vi "Execute Change Boolean Image.vi"(6 "Mouse Position":T1, 8 "User VI Ref":refnum<vi>, 9 "Menu Item Tag Suffix":string, 10 "Remaining Items":refnum<vi>[](array[refnum]), 11 "Affected Items":cluster{"Controls":refnum<vi>[]}) -> (0 "Fail transaction?":bool)   [LabVIEW 2021]
doc: "This VI will set a Boolean type that is input to the control's tag and stays persistent. It marks the data that is used in future application when changing themes.\n\n<b>Original</b>:This VI is part of a plug-in for modifying the LabVIEW shortcut menus. This is the execute VI which is called when the shortcut menu is chosen by the user. It performs the action of the selected menu item."
uses:
  Material-Scheme/Material-Scheme.lvclass
  <vilib>/Utility/miscctls.llb/LVPositionTypeDef.ctl
  Material SubVIs/Material SubVIs.lvlib
panel:
  # "All controls on this panel except \"Affected Items\" have been locked to prevent accidental edits. Changing the control names or types, other than the elements of the \"Affected Items\" cluster will make the VI unusable as a menu plugin.\n\nSee Context Help for each control for details about its use."
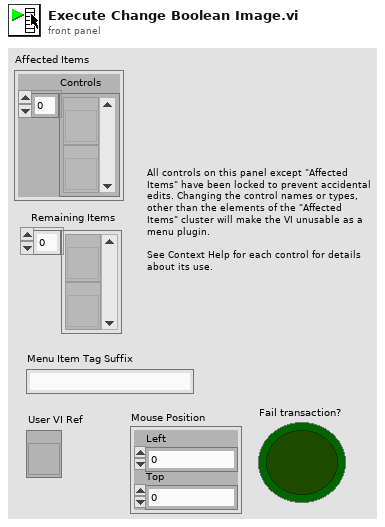
[diagram p1: front panel]
types:
  T1 = typedef "LVPositionTypeDef.ctl" = cluster{"Left":i32, "Top":i32}
  T2 = enum32{"invalid VI type", "Standard VI", "Control VI", "Global VI", "Polymorphic VI", "Configuration VI", "SubSystem", "Facade VI", "Method VI", "Statechart Diagram VI"}
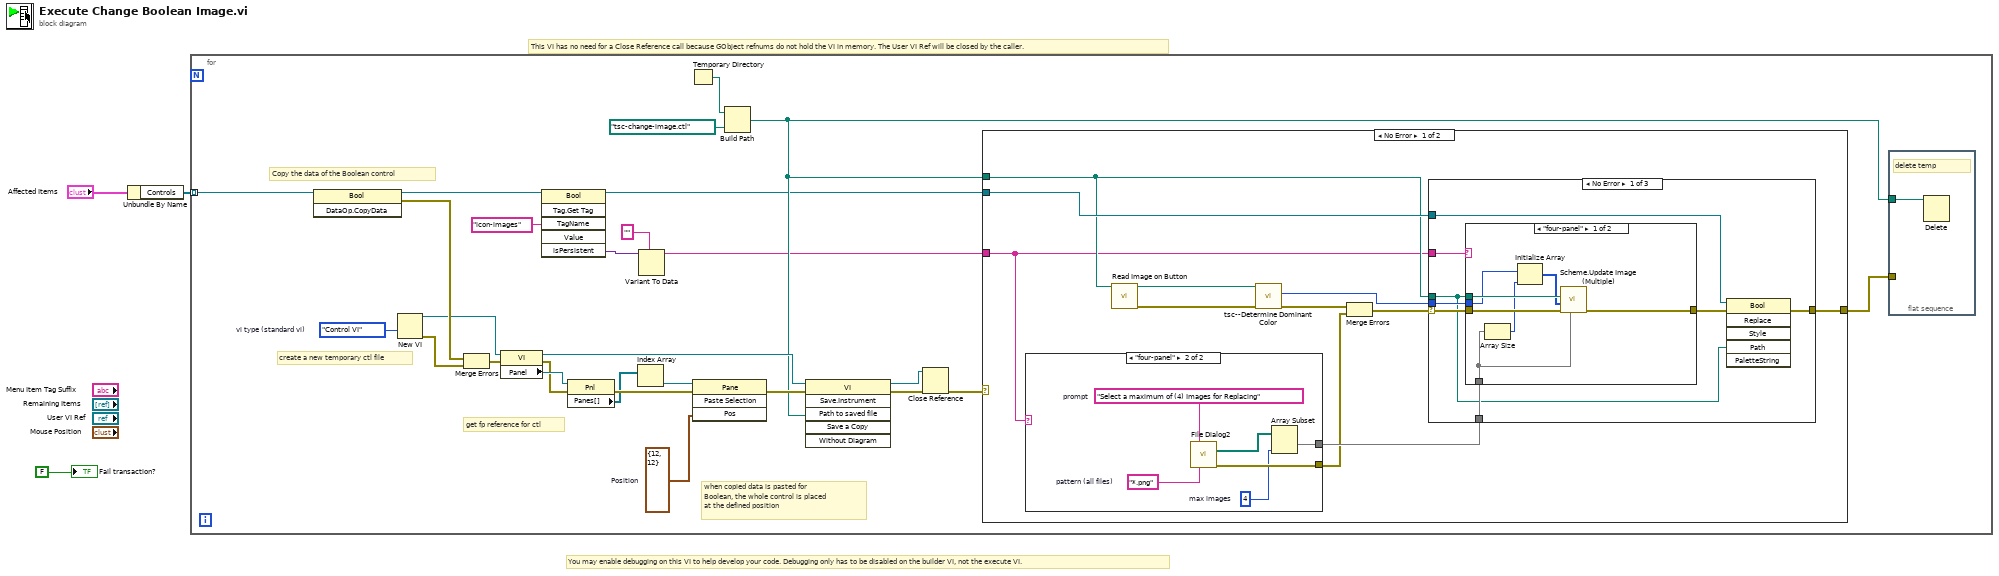
[diagram p0: block diagram]
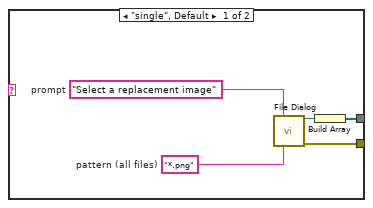
[diagram p2: hidden frame]
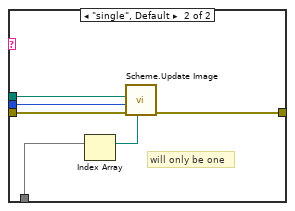
[diagram p3: hidden frame]
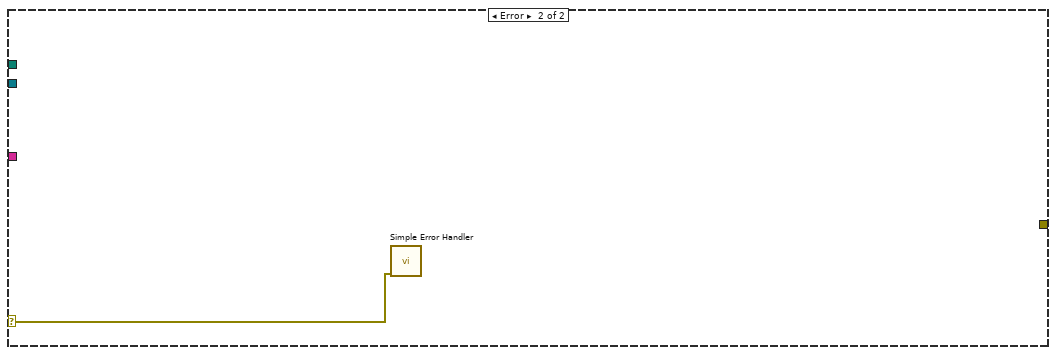
[diagram p6: hidden frame]
diagram:
  # "You may enable debugging on this VI to help develop your code. Debugging only has to be disabled on the builder VI, not the execute VI."
  # "This VI has no need for a Close Reference call because GObject refnums do not hold the VI in memory. The User VI Ref will be closed by the caller."
  n1 = Unbundle By Name("Affected Items") -> ("Controls"=w1:refnum<vi>[])
  n2 = for {
    tunnel: w1 -> [w21] mode=indexing
    w18 = T2."Control VI"  # vi type (standard vi)
    w22 = T1 {"Left"=12, "Top"=12}  # Position
    # "when copied data is pasted for\nBoolean, the whole control is placed \nat the defined position"
    # "get fp reference for ctl"
    # "create a new temporary ctl file"
    # "Copy the data of the Boolean control"
    n3 = invoke class="Bool" method="DataOp.CopyData"(reference=w21) -> (reference out=w11:refnum<vi>, error out=w28:errorcluster)  [unwired: 2 in, 1 out]
    n4 = New VI(9:w18) -> (0:w16:errorcluster, 3:w17:refnum<vi>)  [unwired: 6 in]
    n5 = Merge Errors(w28, w16) -> (w20:errorcluster)
    n6 = property class="VI"(reference=w17, error in=w20) -> (reference out=w26:refnum<vi>, error out=w29:errorcluster, "Panel"=w30:refnum<vi>)
    n7 = invoke class="Bool" method="Tag.Get Tag"(reference=w11, "TagName"="icon-images" ("Tag Name")) -> (reference out=w8:refnum<vi>, "isPersistent"=w6:variant)  [unwired: 4 in, 4 out]
    n8 = property class="Pnl"(reference=w30, error in=w29) -> (error out=w25:errorcluster, "Panes[]"=w24:refnum<vi>[])  [unwired: 1 out]
    n9 = Index Array(array=w24) -> (element=w23:refnum<vi>)  [unwired: 1 in]
    n10 = Variant To Data(type="", Variant=w6) -> (data=w4:string)  [unwired: 1 in, 1 out]
    n11 = Temporary Directory() -> (w15:path)
    n12 = invoke class="Pane" method="Paste Selection"(reference=w23, error in=w25, "Pos"=w22) -> (error out=w27:errorcluster)  [unwired: 1 in, 3 out]
    n13 = Build Path(base path=w15, name or relative path=path "tsc-change-image.ctl") -> (appended path=w9:path)
    n14 = invoke class="VI" method="Save.Instrument"(reference=w26, error in=w27, "Path to saved file"=w9) -> (reference out=w12:refnum<vi>, error out=w19:errorcluster)  [unwired: 3 in, 4 out]
    n15 = Close Reference(reference=w12, error in (no error)=w19) -> (error out=w13:errorcluster)
    n16 = case shown="No Error" w13 {
      selector: w13 -> [_ w76]
      tunnel: w9 -> [w34 _]
      tunnel: w8 -> [w35 _]
      tunnel: [w33 _] -> w10
      tunnel: w4 -> [w32 _]
      frame No Error {
        n17 = case shown="\"four-panel\"" w32 {
          tunnel: [w43 w50] -> w38
          tunnel: [w44 w51] -> w37
          frame "single", Default {
            w47 = "Select a replacement image"  # prompt
            w46 = "*.png"  # pattern (all files)
            n18 = call "File Dialog"("prompt"=w47, "pattern (all files)"=w46) -> ("selected path"=w45:path, "error out"=w44:errorcluster)  [unwired: 10 in, 2 out]
            n19 = Build Array(w45) -> (w43:path[])
          }
          frame "four-panel" {
            w48 = 4  # max images
            w53 = "Select a maximum of (4) Images for Replacing"  # prompt
            w52 = "*.png"  # pattern (all files)
            n20 = call "File Dialog2"("prompt"=w53, "pattern (all files)"=w52) -> ("selected paths"=w49:path[], "error out"=w51:errorcluster)  [unwired: 10 in, 2 out]
            n21 = Array Subset(array=w49, length=w48) -> (w50:path[])  [unwired: 1 in]
          }
        }
        n22 = call "Read Image on Button.vi"("File with Button"=w34) -> ("error out"=w41:errorcluster, "png file out"=w42:path)  [unwired: 9 in]
        n23 = call "tsc--Determine Dominant Color.vi"("error in"=w41, "orig file"=w42) -> ("error out"=w40:errorcluster, "maximum color"=w39:u32)  [unwired: 7 in, 1 out]
        n24 = Merge Errors(w40, w37) -> (w36:errorcluster)
        n25 = case shown="No Error" w36 {
          selector: w36 -> [w59 _ w75]
          tunnel: w39 -> [w61 _ _]
          tunnel: w34 -> [w55 _ _]
          tunnel: w38 -> [w60 _ _]
          tunnel: w35 -> [w58 _ _]
          tunnel: [w56 _ w75] -> w33
          tunnel: w32 -> [w54 _ _]
          frame No Error {
            n26 = case shown="\"four-panel\"" w54 {
              tunnel: w61 -> [w65 w74]
              tunnel: w60 -> [w63 w73]
              tunnel: w59 -> [w68 w72]
              tunnel: [w67 w71] -> w57
              tunnel: w55 -> [w66 w70]
              frame "four-panel" {
                n27 = Array Size(array=w63) -> (size(s)=w62:i32)
                n28 = Initialize Array(w65, w62) -> (w64:u32[])
                n29 = call "Scheme.Update Image (Multiple).vi"("Replace Image"=w63, "error in"=w68, "New Color"=w64, "New Control"=w66) -> ("error out"=w67:errorcluster)  [unwired: 5 in, 2 out]
              }
              frame "single", Default {
                # "will only be one"
                n30 = Index Array(array=w73) -> (element=w69:path)  [unwired: 1 in]
                n31 = call "Scheme.Update Image.vi"("Replace Image"=w69, "error in"=w72, "New Color"=w74, "New Control"=w70) -> ("error out"=w71:errorcluster)  [unwired: 6 in, 1 out]
              }
            }
            n32 = invoke class="Bool" method="Replace"(reference=w58, error in=w57, "Path"=w55) -> (error out=w56:errorcluster)  [unwired: 3 in, 5 out]
          }
          frame Error {
          }
          frame Default {
          }
        }
      }
      frame Error {
        n33 = call <vilib>:"Simple Error Handler.vi"("error in (no error)"=w76) -> ()  [unwired: 4 in, 5 out]
      }
    }
    n34 = flat-sequence {
      tunnel: w10 -> [_]
      tunnel: w9 -> [w31]
      frame #0 {
        # "delete temp"
        n35 = Delete(path (use dialog)=w31) -> ()  [unwired: 4 in, 3 out]
      }
    }
  }
  "Fail transaction?" <- FALSE ("Fail transaction?")
